vi "Format Columns.vi"(6 "Delimiter":string, 8 "Column 3":string, 9 "Column 2":string, 10 "Column 1":string, 11 "Last String":string) -> (3 "Result String":string)   [LabVIEW 2025]
doc: "This VI builds a line of text with three columns separated by a delimiter, finishing the string with an \"End of line\"."
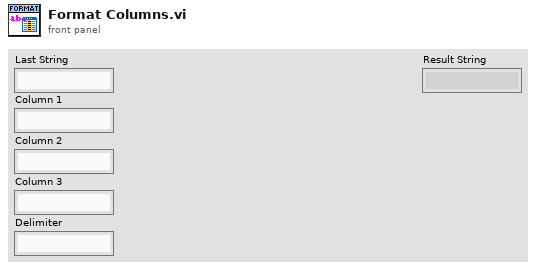
[diagram p1: front panel]
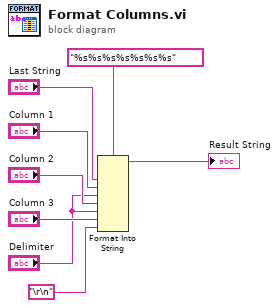
[diagram p0: block diagram]
diagram:
  n1 = Format Into String(format string="%s%s%s%s%s%s%s", "Last String", "Column 1", "Delimiter", "Column 2", "Delimiter", "Column 3", "\r\n") -> (resulting string=→"Result String":string)  [unwired: 2 in, 1 out]
